vi "Write Waiting to Order Dispatcher.vi"(8 "error in (no error)":errorcluster, 10 "Actor Framework.lvlib:Message Enqueuer":refnum<class "Message Enqueuer.lvclass">, 11 "Customer in":refnum<class "Customer.lvclass">) -> (0 "error out":errorcluster, 3 "Customer out":refnum<class "Customer.lvclass">)   [LabVIEW 2023, in "Customer.lvlib" / "Customer.lvclass"]
doc: "Sets the Waiting to Order dispatcher enqueuer reference.\n\nThis dispatcher is analogous to the line of customers waiting in the shop for the next available cashier."
uses:
  Customer.lvclass
  <vilib>/ActorFramework/Message Enqueuer/Message Enqueuer.lvclass
  Customer.lvclass/Customer.ctl
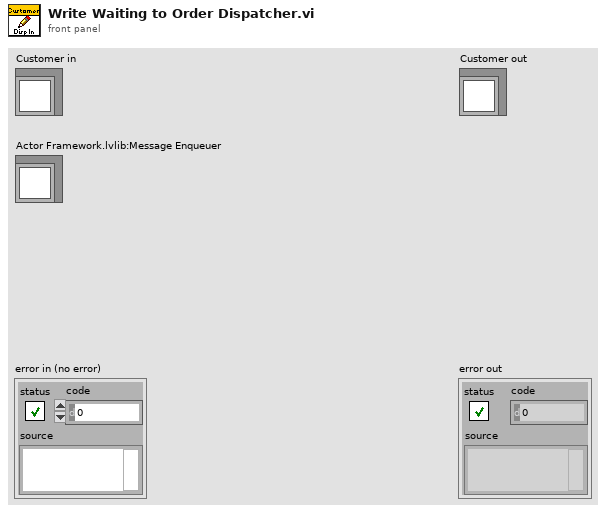
[diagram p1: front panel]
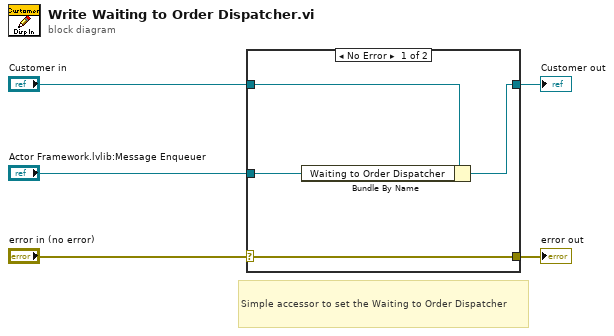
[diagram p0: block diagram]
diagram:
  # "Simple accessor to set the Waiting to Order Dispatcher"
  n1 = case shown="No Error" "error in (no error)" {
    selector: "error in (no error)" -> [w9 w10]
    tunnel: [w9 w10] -> w4
    tunnel: [w7 w11] -> w2
    tunnel: "Customer in" -> [w8 w11]
    tunnel: "Actor Framework.lvlib:Message Enqueuer" -> [w6 _]
    frame No Error {
      n2 = Bundle By Name(cluster=w8, "Waiting to Order Dispatcher"=w6) -> (w7:refnum<class "Customer.lvclass">)
    }
    frame Error {
    }
  }
  "error out" <- w4
  "Customer out" <- w2
